vi "TagBus_Cluster to TagBus Index.vi"(7 "Clust Refnum":refnum<vi>, 10 "Process Name Modifier":string, 11 "TagBus":refnum<class "TagBus.lvclass">) -> (2 "Index Array":i32[](array[numeric]), 3 "TagBus out":refnum<class "TagBus.lvclass">)   [LabVIEW 2015, in "TagBus.lvclass"]
uses:
  TagBus.lvclass
  TagBus.lvclass/TagBus.ctl
  <vilib>/NI/Tag Bus/tag/Data Type.ctl
  <vilib>/Utility/Data Type/NI_Data Type.lvlib
  <vilib>/NI/Tag Bus/tag/tag descriptor.lvclass
  <vilib>/NI/Tag Bus/dictionary/data dictionary.lvclass
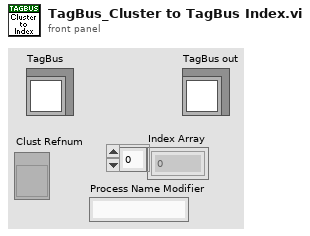
[diagram p1: front panel]
types:
  T1 = typedef "tag bus.lvlib/tag descriptor.lvclass/Data Type.ctl" = enum16{"Double", "Single", "I64", "I32", "I16", "I8", "U64", "U32", "U16", "U8", "Boolean", "String", "Array of Double", "Array of Single", "Array of I64", "Array of I32", "Array of I16", "Array of I8", "Array of U64", "Array of U32", "Array of U16", "Array of U8", "Array of Boolean", "Array of String"}
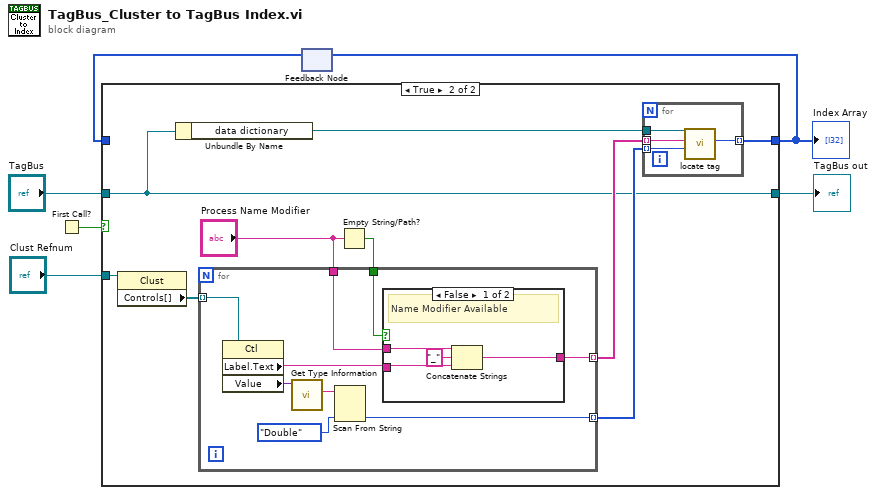
[diagram p0: block diagram]
diagram:
  n1 = First Call?() -> (First Call?: T/F=w5:bool)
  n2 = feedback #1() -> (w4:i32[])  [unwired: 1 in]
  n3 = case shown="True" w5 {
    tunnel: "TagBus" -> [w7 w9]
    tunnel: [w8 w17] -> w6
    tunnel: w4 -> [w8 _]
    tunnel: [w7 w9] -> w2
    tunnel: "Clust Refnum" -> [_ w15]
    frame False {
    }
    frame True {
      n4 = property class="Clust"(reference=w15) -> ("Controls[]"=w14:refnum<vi>[])  [unwired: 1 in, 2 out]
      n5 = Unbundle By Name(w9) -> ("data dictionary"=w16:refnum<class "data dictionary.lvclass">)
      n6 = Empty String/Path?(string/path="Process Name Modifier") -> (empty?=w10:bool)
      n7 = for {
        tunnel: w14 -> [w26] mode=indexing
        tunnel: [w22] -> w12 mode=indexing
        tunnel: [w20] -> w13 mode=indexing
        tunnel: "Process Name Modifier" -> [w19]
        tunnel: w10 -> [w18]
        n8 = property class="Ctl"(reference=w26) -> ("Label.Text"=w21:string, "Value"=w25:variant)  [unwired: 1 in, 2 out]
        n9 = call <vilib>:"Get Type Information.vi"("Variant"=w25) -> ("Name"=w23:string)  [unwired: 6 in, 4 out]
        n10 = Scan From String(input string=w23, default 1=Data_Type."Double" ("data type")) -> (output 1=w22:T1)  [unwired: 3 in, 3 out]
        n11 = case shown="False" w18 {
          tunnel: w21 -> [w30 w31]
          tunnel: [w29 w31] -> w20
          tunnel: w19 -> [w27 _]
          frame False {
            # "Name Modifier Available"
            n12 = Concatenate Strings(w27, "_" ("string"), w30) -> (w29:string)
          }
          frame True {
          }
        }
      }
      n13 = for {
        tunnel: w16 -> [w35]
        tunnel: w13 -> [w34] mode=indexing
        tunnel: [w33] -> w17 mode=indexing
        tunnel: w12 -> [w32] mode=indexing
        n14 = call <vilib>:"locate tag.vi"("data type"=w32, "name"=w34, "data dictionary in"=w35) -> ("index"=w33:i32)  [unwired: 6 in, 2 out]
      }
    }
  }
  "Index Array" <- w6
  "TagBus out" <- w2
  n15 = feedback-in #1(w6) -> ()
